vi "Mark_CreateAverageFromBE.vi"(7 "Dilate Length":i32=200, 8 "error in (no error)":errorcluster, 10 "Variables":string[](array[string]), 11 "ExpData in":refnum<class "ExpData.lvclass">) -> (0 "error out":errorcluster, 1 "Std":dbl[][](array[numeric]), 2 "Mean":dbl[][](array[numeric]), 3 "ExpData out":refnum<class "ExpData.lvclass">, 4 "ColHeaders":string[](array[string]))   [LabVIEW 2015, in "ExpData.lvclass"]
uses:
  ExpData.lvclass
  CustomVIs/CustomVI.lvlib
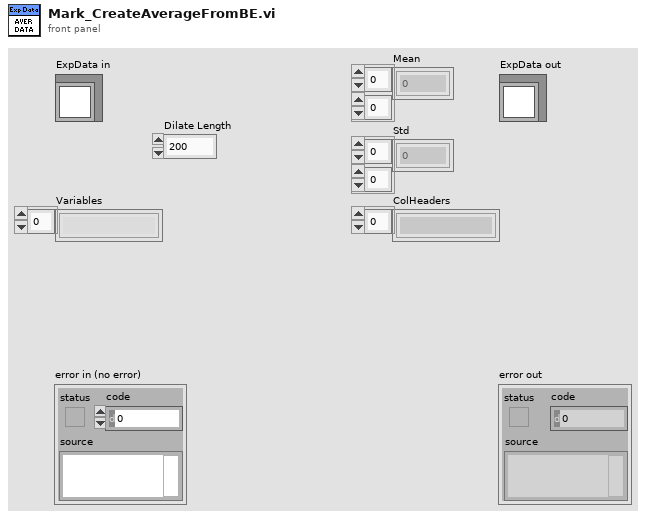
[diagram p1: front panel]
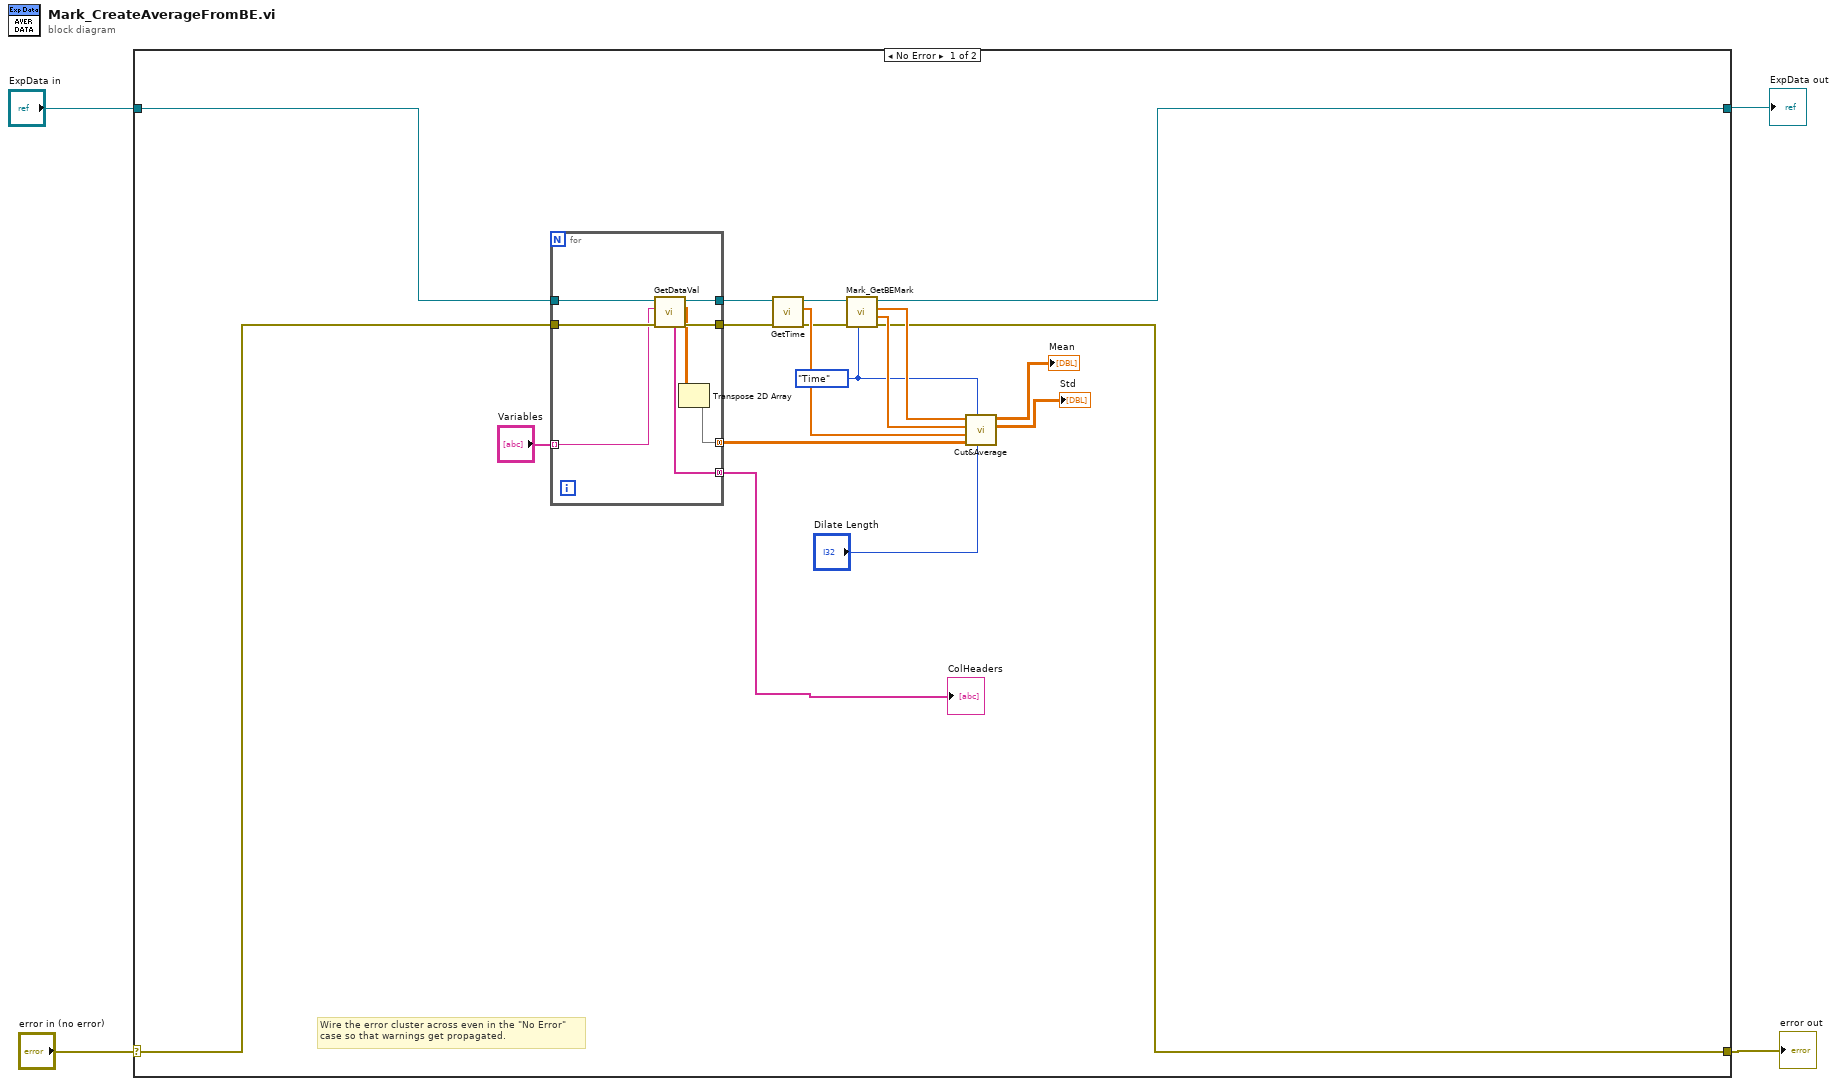
[diagram p0: block diagram]
diagram:
  n1 = case shown="No Error" "error in (no error)" {
    selector: "error in (no error)" -> [w14 w32]
    tunnel: [w13 w32] -> w3
    tunnel: [w11 w31] -> w1
    tunnel: "ExpData in" -> [w12 w31]
    frame No Error {
      w9 = enum16{"Time", "Percentage", "Index"}."Time" ("Type (Time)")
      # "Wire the error cluster across even in the \"No Error\"\ncase so that warnings get propagated."
      n2 = for {
        tunnel: [w30] -> w17
        tunnel: [w29] -> w16
        tunnel: w12 -> [w28]
        tunnel: w14 -> [w27]
        tunnel: "Variables" -> [w26] mode=indexing
        tunnel: [w23] -> w5 mode=concatenating
        tunnel: [w24] -> w6 mode=concatenating
        n3 = call "GetDataVal.vi"("error in (no error)"=w27, "Name"=w26, "CarexMData in"=w28) -> ("error out"=w30:errorcluster, "Data"=w25:dbl[][], "CarexMData out"=w29:refnum<class "ExpData.lvclass">, "ColHeaders"=w24:string[])  [unwired: 5 in]
        n4 = Transpose 2D Array(2D array=w25) -> (transposed array=w23:dbl[][])
      }
      "ColHeaders" <- w6
      n5 = call "GetTime.vi"("error in (no error)"=w17, "CarexMData in"=w16) -> ("error out"=w18:errorcluster, "Time"=w20:dbl[], "CarexMData out"=w19:refnum<class "ExpData.lvclass">)  [unwired: 7 in]
      n6 = call "Mark_GetBEMark.vi"("Type (Time)"=w9, "error in (no error)"=w18, "ExpData In"=w19) -> ("error out"=w13:errorcluster, "End"=w21:dbl[], "Begin"=w22:dbl[], "ExpData Out"=w11:refnum<class "ExpData.lvclass">)  [unwired: 4 in, 1 out]
      n7 = call "Cut&Average.vi"("Dilate Length (200)"="Dilate Length", "Input Type (Time)"=w9, "Data"=w5, "Time"=w20, "End"=w21, "Begin"=w22) -> ("Std"=→"Std":dbl[][], "Mean"=→"Mean":dbl[][])  [unwired: 4 out]
    }
    frame Error {
    }
  }
  "error out" <- w3
  "ExpData out" <- w1
